vi "Average Readings U16.vi"(9 "Input Array Data U16":u16[](array[numeric]), 11 "# of Points":u16) -> (3 "Average":u16)   [LabVIEW 2010]
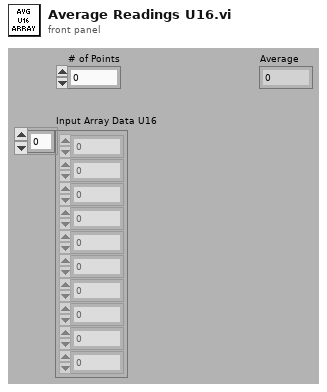
[diagram p1: front panel]
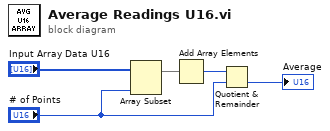
[diagram p0: block diagram]
diagram:
  n1 = Array Subset(array="Input Array Data U16", length="# of Points") -> (w4:u16[])  [unwired: 1 in]
  n2 = Add Array Elements(numeric array=w4) -> (sum=w3:u16)
  n3 = Quotient & Remainder(x=w3, y="# of Points") -> (floor(x/y)=→"Average":u16)  [unwired: 1 out]
